vi "select energy.vi"(8 "Error In":errorcluster, 9 "List ROI in":dbl[][](array[numeric]), 10 "List Peak":string[][](table)=[["0", "0.738169", "8216.078017"], ["1", "1.925791", "11797.605609"], ["2", "2.296686", "59445.586632"], ["3", "2.951953", "7958.809520"], ["4", "3.301930", "5536.954047"], ["5", "3.693063", "592063.911968"], ["6", "4.012579", "88599.650063"], ["7", "5.456304", "6013.116723"], ["8", "5.905392", "7038.874622"], ["9", "6.404196", "22471.618393"], ["10", "7.049745", "8038.961303"], ["11", "7.336853", "5649.863203"], ["12", "7.978842", "3458.992769"], ["13", "8.617482", "7301.160509"], ["14", "9.554502", "1097.160220"], ["15", "10.523191", "20487.327187"], ["16", "11.054270", "2935.510385"], ["17", "11.234771", "2776.270069"], ["18", "12.573155", "28067.247871"], ["19", "13.048495", "7100.524309"], ["20", "13.060056", "7093.993228"], ["21", "13.100857", "7126.608473"], ["22", "13.283153", "7227.068614"], ["23", "14.060270", "10970.472713"], ["24", "14.659482", "8813.189447"], ["25", "15.701110", "4886.263831"], ["26", "16.589220", "151655.425908"], ["27", "17.295466", "73726.613413"], ["28", "18.547307", "16625.597400"], ["29", "19.386897", "11325.808412"], ["30", "23.791659", "1504.095156"], ["31", "24.239552", "1887.308691"], ["32", "24.942128", "13678.898904"]], 11 "Spectrum":cluster{"Channels":dbl[], "Intensity":dbl[]}[](graph)) -> (0 "Error Out":errorcluster, 1 "List ROI out":dbl[][](array[numeric]), 2 "Peak Position":cluster{"Array":dbl[], "Array":dbl[]}, 3 "Elements":string[][](table))   [LabVIEW 2023]
uses:
  <vilib>/Utility/miscctls.llb/LVRowAndColumnTypeDef.ctl
  06da3617-9ec4-42f1-9290-0e5eb46bbf30.vi
  84818e8e-7348-432d-a6d3-ef5b80d9228f.vi
  8a708491-6dff-4872-9c8c-723543562d7f.vi
  <vilib>/Utility/Data Type/Get Array Information.vi
  <vilib>/Utility/Data Type/Get Type Information.vi
  queue/Front Panel Message Queue.lvlib
panel:
  in  "list peak vs energy":bool
  out "reference list peak":refnum<vi>
  in  "Add":bool
  in  "ordinate":u16(ring) items=["Linear", "Logarithmic"]
  in  "doubt":bool
  in  "reset":bool
  out "List In":cluster{"Channels":dbl[], "Intensity":dbl[]}
  out "Data In":cluster{"Channels":dbl[], "Intensity":dbl[]}
  out "Element Position Peaks":dbl[][](array[numeric])
  out "Best Match":string[][](table)
  in  "exit":bool
  # "?"
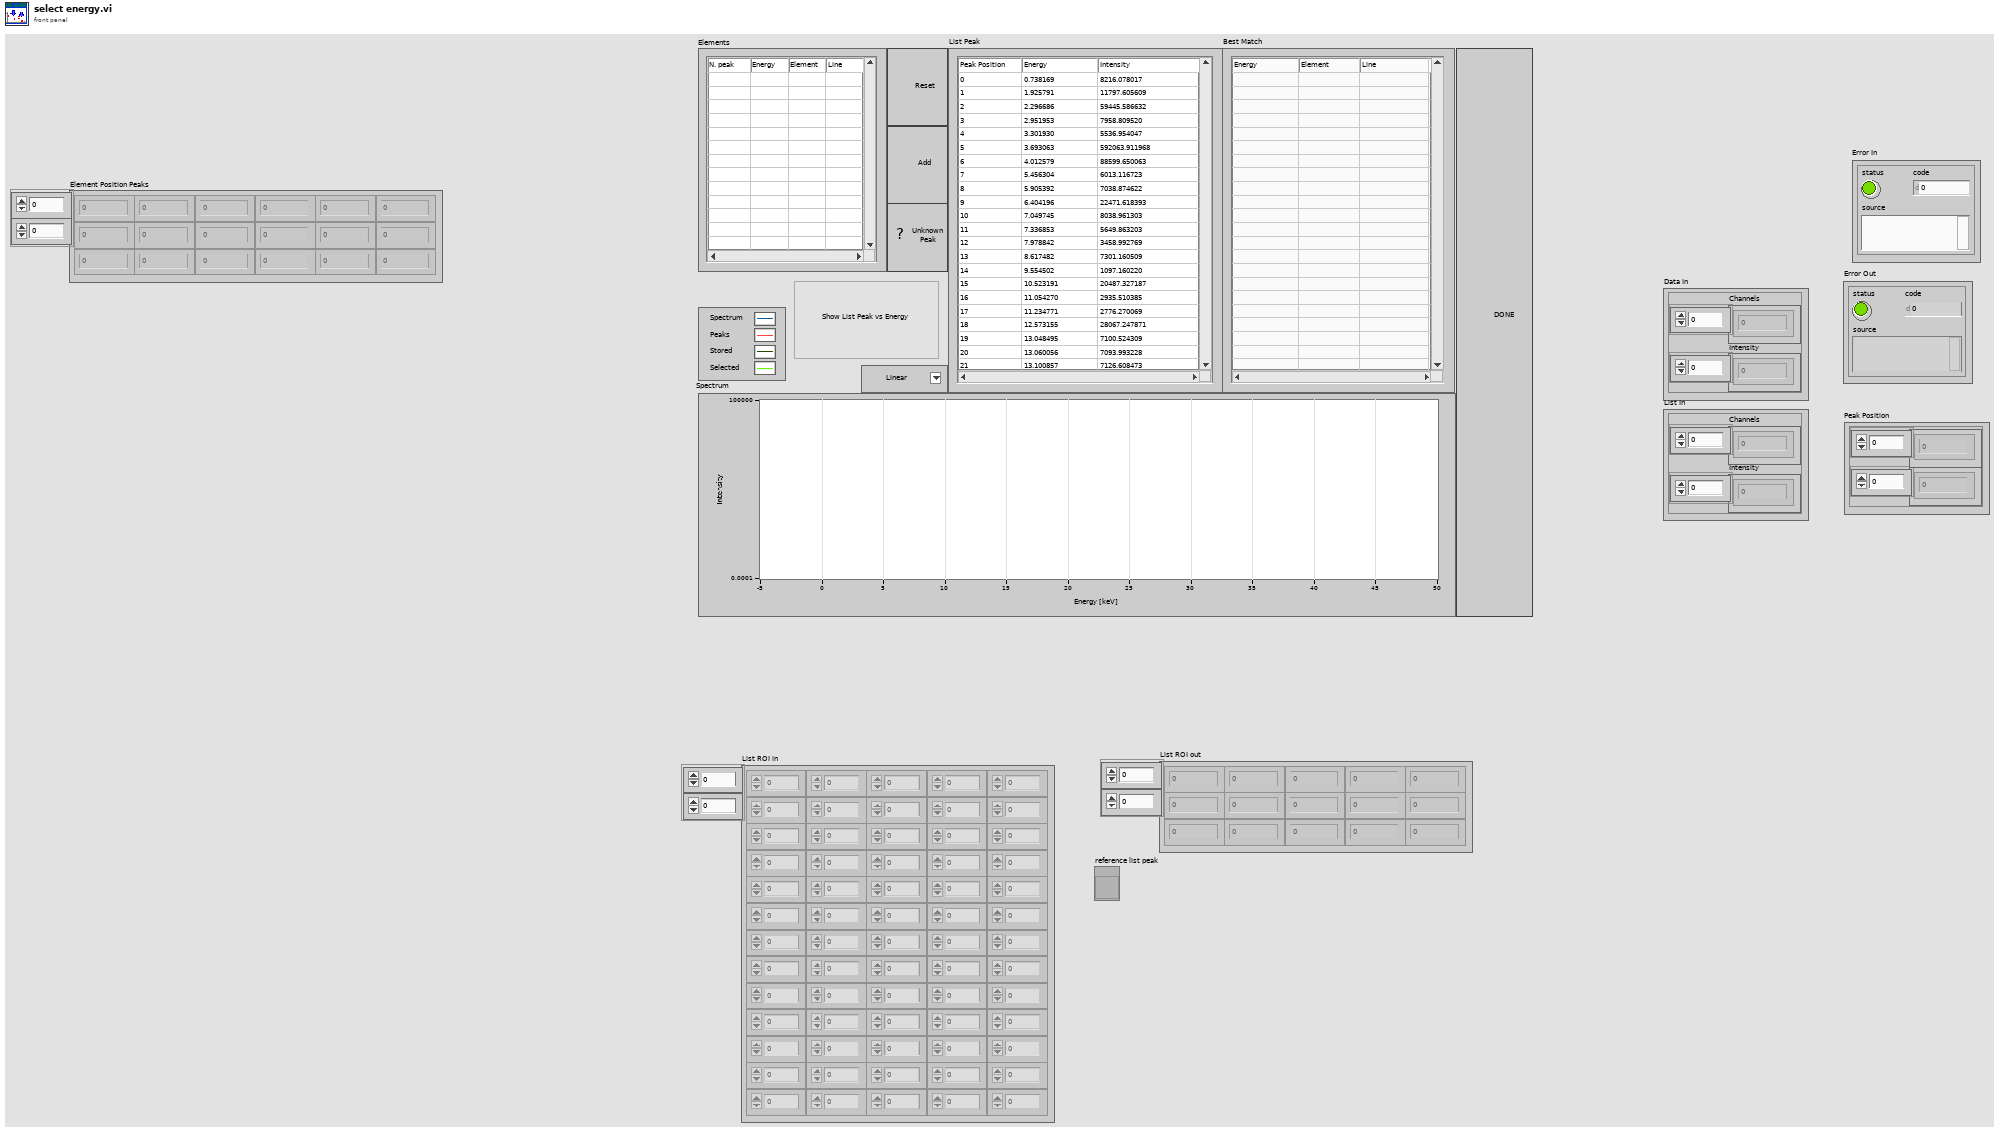
[diagram p1: front panel]
types:
  T1 = typedef "Front Panel Message Queue.lvlib/load Message Queues.ctl" = cluster{"Main":refnum<queue>}
  T2 = enum32{"Invalid", "Standard", "Closed", "Hidden", "Minimized", "Maximized"}
  T3 = typedef "LVRowAndColumnTypeDef.ctl" = cluster{"Row":i32, "Column":i32}
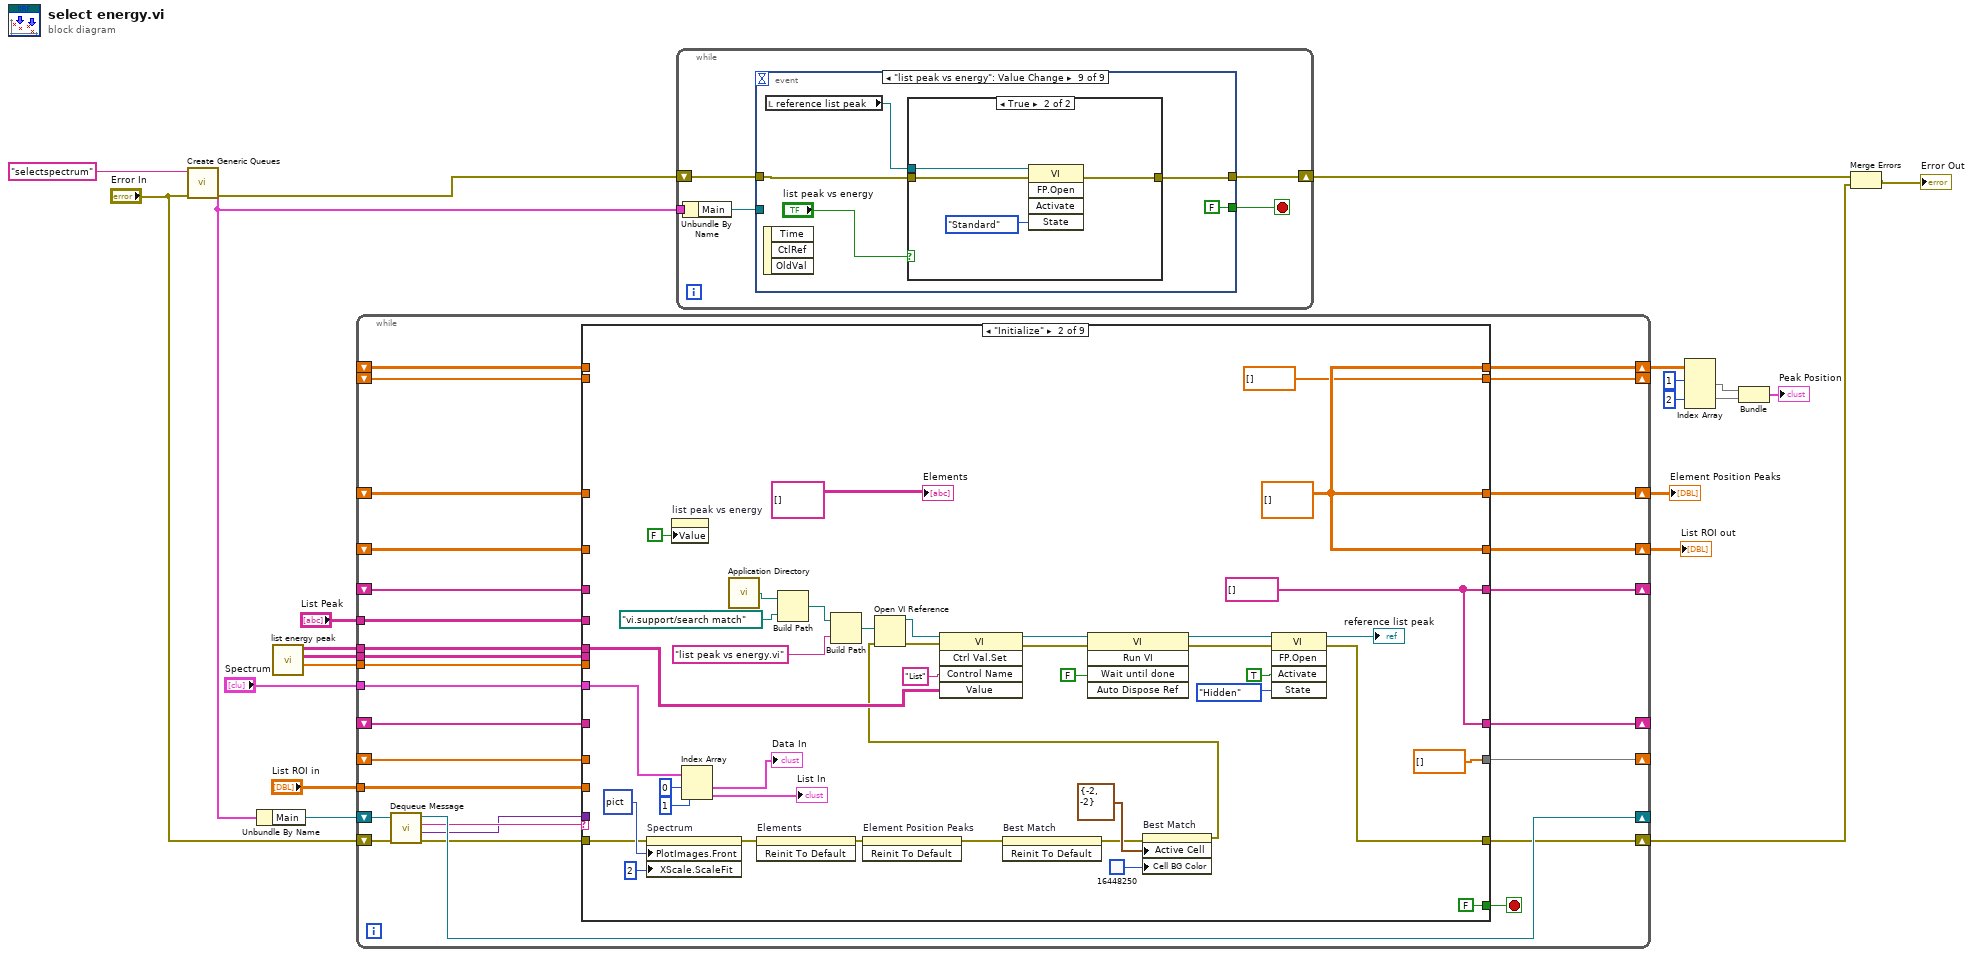
[diagram p0: block diagram]
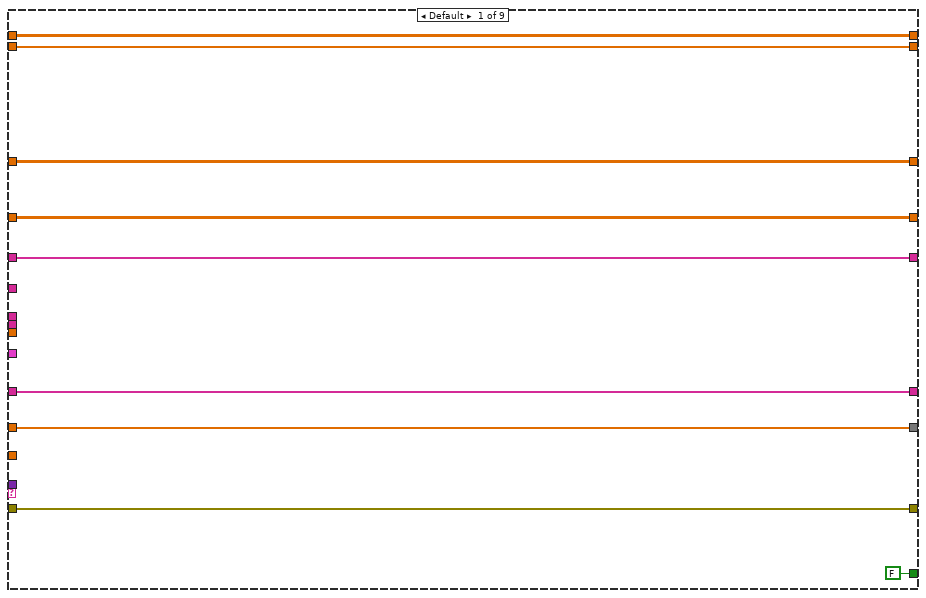
[diagram p2: hidden frame]
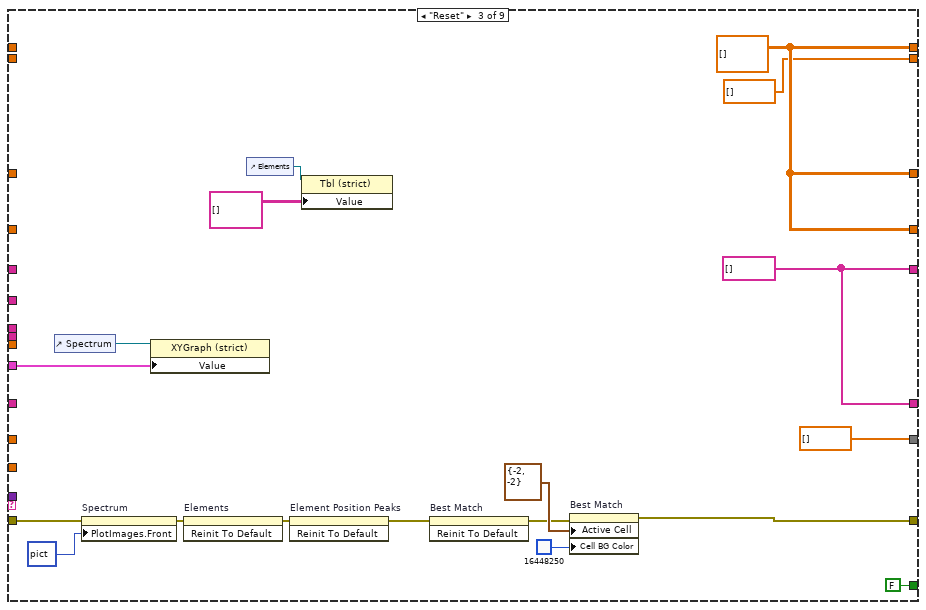
[diagram p3: hidden frame]
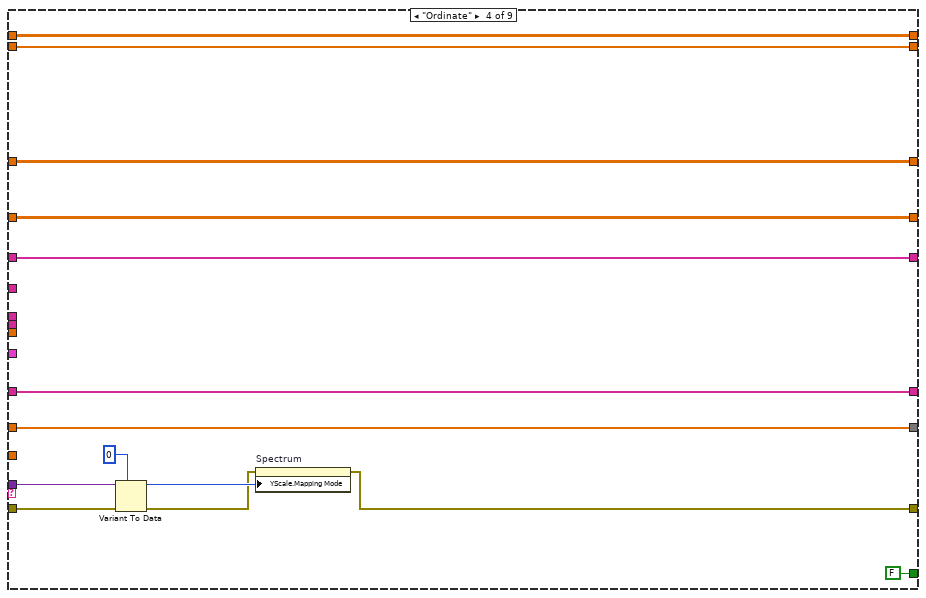
[diagram p4: hidden frame]
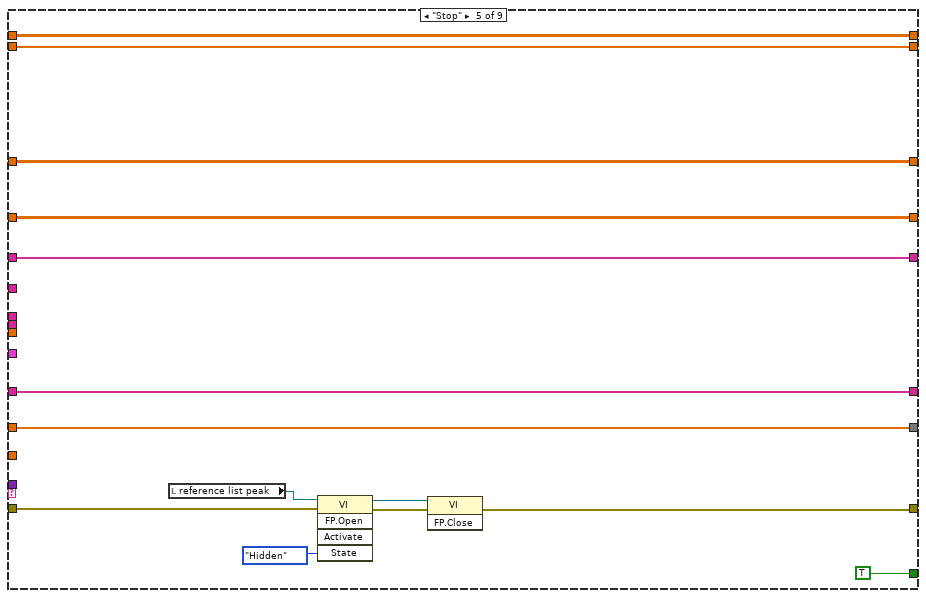
[diagram p5: hidden frame]
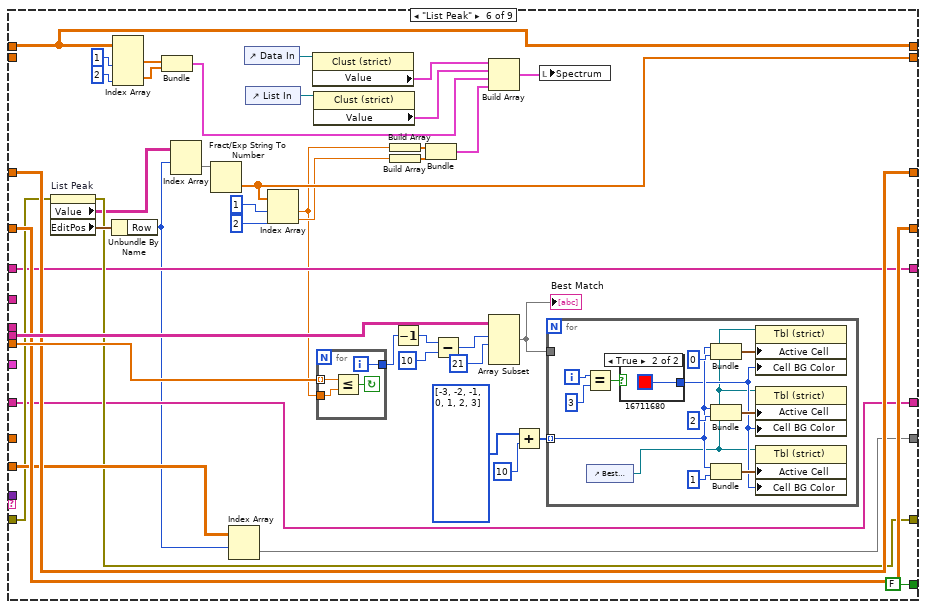
[diagram p6: hidden frame]
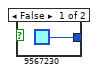
[diagram p7: hidden frame]
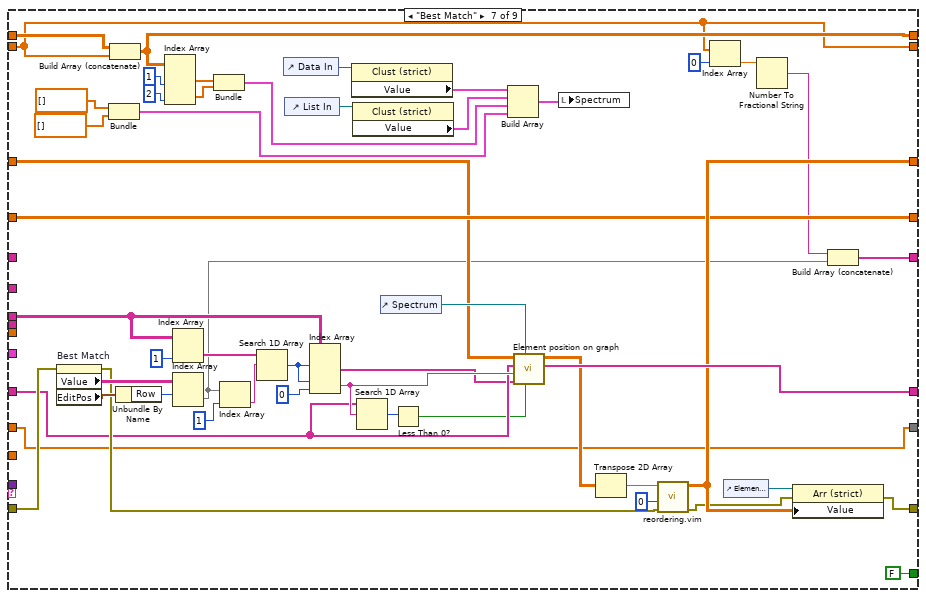
[diagram p8: hidden frame]
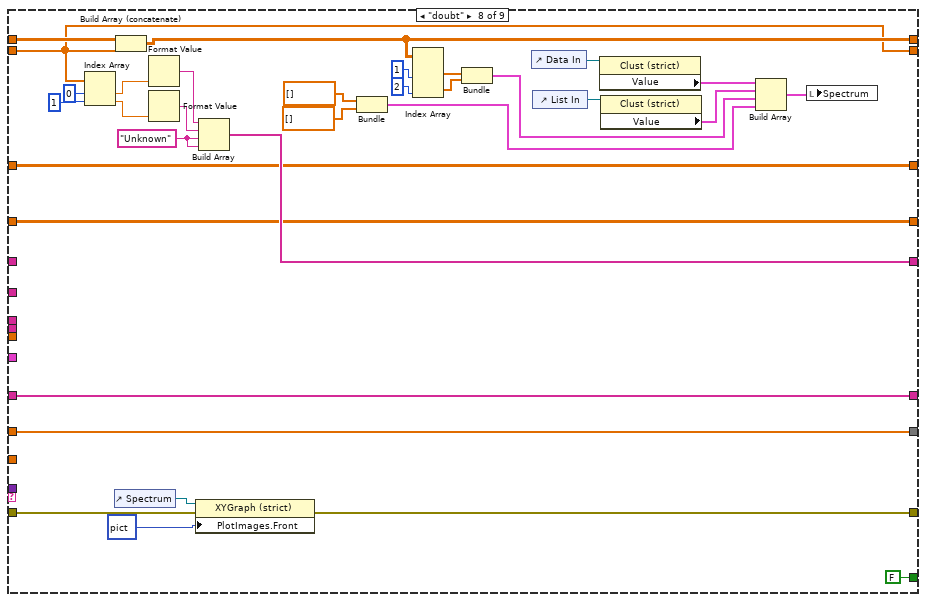
[diagram p9: hidden frame]
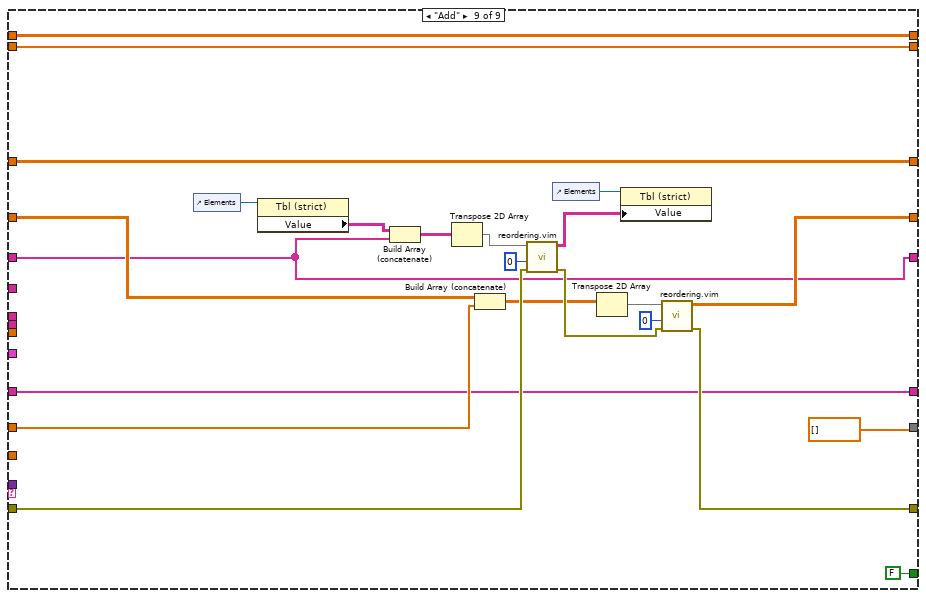
[diagram p10: hidden frame]
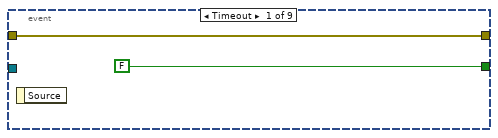
[diagram p11: hidden frame]
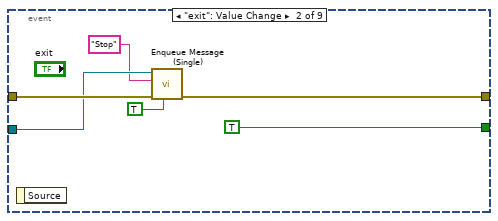
[diagram p12: hidden frame]
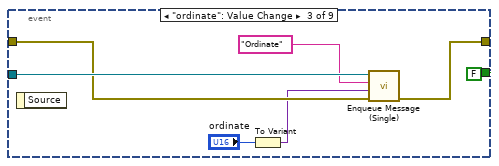
[diagram p13: hidden frame]
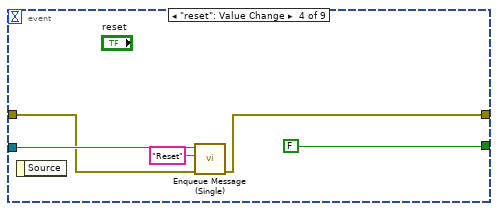
[diagram p14: hidden frame]
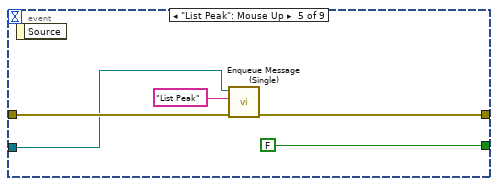
[diagram p15: hidden frame]
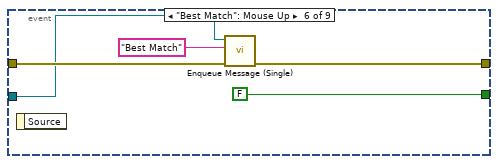
[diagram p16: hidden frame]
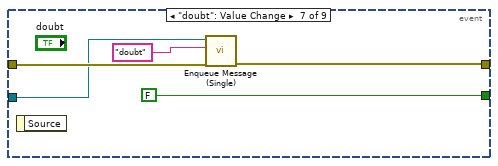
[diagram p17: hidden frame]
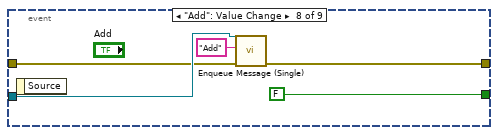
[diagram p18: hidden frame]
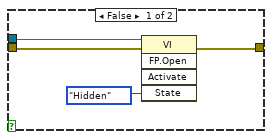
[diagram p19: hidden frame]
diagram:
  n1 = call "Create Generic Queues.vi"("error in (no error)"="Error In", "name"="selectspectrum") -> ("error out"=w21:errorcluster, "Message Queues"=w14:T1)  [unwired: 8 in]
  n2 = Unbundle By Name(w14) -> ("Main"=w19:refnum<queue>)
  n3 = call "list energy peak.vi"() -> ("Energies Ordered"=w15:dbl[], "List Ordered"=w16:string[][], "List"=w17:string[][])  [unwired: 6 in, 3 out]
  n4 = while {
    shift-right: [w45] -> w2
    shift-left: "Error In" -> [w50]
    shift-right: [w48] -> _
    shift-left: w19 -> [w49]
    tunnel: "Spectrum" -> [w47]
    tunnel: w17 -> [w23]
    tunnel: w16 -> [w25]
    tunnel: w15 -> [w26]
    shift-right: [w41] -> _
    shift-left: _ -> [w40]
    shift-right: [w39] -> w10
    shift-left: _ -> [w38]
    shift-right: [w37] -> w11
    shift-left: _ -> [w32]
    shift-right: [w36] -> w5
    shift-left: _ -> [w33]
    shift-right: [w35] -> _
    shift-left: _ -> [w34]
    shift-right: [w31] -> _
    shift-left: _ -> [w28]
    shift-right: [w30] -> _
    shift-left: _ -> [w29]
    tunnel: "List Peak" -> [w27]
    tunnel: "List ROI in" -> [w24]
    stop <- w43 stop-if-true
    n5 = call "Dequeue Message.vi"("error in (no error)"=w50, "Message Queue"=w49) -> ("error out"=w46:errorcluster, "Message Data"=w42:variant, "Message"=w44:string, "dup Message Queue"=w48:refnum<queue>)  [unwired: 5 in, 1 out]
    n6 = case shown="\"Initialize\"" w44 {
      tunnel: w46 -> [w58 w92 w110 w130 w136 w158 w240 w279 w305]
      tunnel: w47 -> [_ w89 w106 _ _ _ _ _ _]
      tunnel: [w58 w69 w109 w127 w132 w159 w219 w277 w301] -> w45
      tunnel: [FALSE FALSE FALSE FALSE TRUE FALSE FALSE FALSE FALSE] -> w43
      tunnel: w42 -> [_ _ _ w125 _ _ _ _ _]
      tunnel: [w57 dbl[] [] dbl[] [] w124 w144 w152 w228 w260 w292] -> w41
      tunnel: w40 -> [w57 _ _ w124 w144 _ w228 w260 w292]
      tunnel: [w53 w85 w105 w123 w143 w177 w253 w261 w291] -> w39
      tunnel: w38 -> [w53 _ _ w123 w143 w177 w256 w289 w291]
      tunnel: [w54 w85 w105 w122 w142 w166 w221 w273 w293] -> w37
      tunnel: [w55 w85 w105 w121 w141 w167 w216 w274 w298] -> w36
      tunnel: [w56 dbl[] [] dbl[] [] w120 w140 w164 w217 w276 dbl[] []] -> w35
      tunnel: w34 -> [w56 _ _ w120 w140 _ w217 w276 w299]
      tunnel: w33 -> [w55 _ _ w121 w141 w167 w216 w274 w297]
      tunnel: w32 -> [w54 _ _ w122 w142 w166 w215 w273 w293]
      tunnel: [w52 w83 w101 w119 w139 w157 w229 w281 w294] -> w31
      tunnel: [w51 w83 w101 w118 w138 w156 w227 w275 w295] -> w30
      tunnel: w29 -> [w51 _ _ w118 w138 w156 w213 w275 w295]
      tunnel: w28 -> [w52 _ _ w119 w139 w157 _ _ w294]
      tunnel: w27 -> [_ _ _ _ _ _ _ _ _]
      tunnel: w26 -> [_ _ _ _ _ w174 _ _ _]
      tunnel: w25 -> [_ _ _ _ _ w168 _ _ _]
      tunnel: w24 -> [_ _ _ _ _ w165 _ _ _]
      tunnel: w23 -> [_ w72 _ _ _ _ w235 _ _]
      frame Default {
      }
      frame "Initialize" {
        w83 = string[] [] ("Value")
        w85 = dbl[][] []
        n7 = property on="Spectrum" class="XYGraph (strict)"(error in=w92, "PlotImages.Front"=picture data[5B] ("line to place"), "XScale.ScaleFit"=u8 2 ("X Scale.Scale Fit")) -> (error out=w99:errorcluster)  [unwired: 1 in, 1 out]
        n8 = property on="list peak vs energy" class="Bool (strict)"("Value"=FALSE ("list peak")) -> ()  [unwired: 2 in, 2 out]
        n9 = Index Array(array=w89, index #1=0 ("index"), index #2=1 ("index")) -> (element #1=→"Data In":cluster{"Channels":dbl[], "Intensity":dbl[]}, element #2=→"List In":cluster{"Channels":dbl[], "Intensity":dbl[]})
        n10 = call <vilib>:"Application Directory.vi"() -> ("Application Directory"=w79:path)
        n11 = invoke on="Elements" class="Tbl (strict)" method="Reinit To Default"(error in=w99) -> (error out=w93:errorcluster)  [unwired: 2 in, 2 out]
        n12 = Build Path(base path=w79, name or relative path=path "vi.support/search match") -> (appended path=w74:path)
        n13 = Build Path(base path=w74, name or relative path="list peak vs energy.vi") -> (appended path=w76:path)
        n14 = invoke on="Element Position Peaks" class="Arr (strict)" method="Reinit To Default"(error in=w93) -> (error out=w97:errorcluster)  [unwired: 2 in, 2 out]
        n15 = invoke on="Best Match" class="Tbl (strict)" method="Reinit To Default"(error in=w97) -> (error out=w94:errorcluster)  [unwired: 2 in, 2 out]
        n16 = property on="Best Match" class="Tbl (strict)"(error in=w94, "Active Cell"=T3 {"Row"=-2, "Column"=-2} ("Active Cell:Active Cell"), "Cell BG Color"=u32 16448250) -> (error out=w71:errorcluster)  [unwired: 1 in, 1 out]
        n17 = Open VI Reference(vi path=w76, error in (no error)=w71) -> (vi reference=w66:refnum<vi>, error out=w65:errorcluster)  [unwired: 4 in]
        n18 = invoke class="VI" method="Ctrl Val.Set"(reference=w66, error in=w65, "Control Name"="List", "Value"=w72) -> (reference out=w64:refnum<vi>, error out=w63:errorcluster)  [unwired: 1 in, 3 out]
        n19 = invoke class="VI" method="Run VI"(reference=w64, error in=w63, "Wait until done"=FALSE ("Wait Until Done")) -> (reference out=w61:refnum<vi>, error out=w62:errorcluster)  [unwired: 2 in, 3 out]
        n20 = invoke class="VI" method="FP.Open"(reference=w61, error in=w62, "Activate"=TRUE ("Activate?"), "State"=T2."Hidden") -> (reference out=→"reference list peak":refnum<vi>, error out=w69:errorcluster)  [unwired: 1 in, 3 out]
        "Elements" <- string[][] [] ("Data Out")
      }
      frame "Reset" {
        w101 = string[] [] ("Value")
        w105 = dbl[][] []
        n21 = control-ref of="Spectrum"() -> (w107:refnum<vi>)
        n22 = property on="Spectrum" class="XYGraph (strict)"(error in=w110, "PlotImages.Front"=picture data[5B] ("line to place")) -> (error out=w117:errorcluster)  [unwired: 1 in, 1 out]
        n23 = property class="XYGraph (strict)"(reference=w107, "Value"=w106) -> ()  [unwired: 1 in, 2 out]
        n24 = invoke on="Elements" class="Tbl (strict)" method="Reinit To Default"(error in=w117) -> (error out=w111:errorcluster)  [unwired: 2 in, 2 out]
        n25 = control-ref of="Elements"() -> (w103:refnum<vi>)
        n26 = invoke on="Element Position Peaks" class="Arr (strict)" method="Reinit To Default"(error in=w111) -> (error out=w115:errorcluster)  [unwired: 2 in, 2 out]
        n27 = property class="Tbl (strict)"(reference=w103, "Value"=string[][] [] ("Data Out")) -> ()  [unwired: 1 in, 2 out]
        n28 = invoke on="Best Match" class="Tbl (strict)" method="Reinit To Default"(error in=w115) -> (error out=w112:errorcluster)  [unwired: 2 in, 2 out]
        n29 = property on="Best Match" class="Tbl (strict)"(error in=w112, "Active Cell"=T3 {"Row"=-2, "Column"=-2} ("Active Cell:Active Cell"), "Cell BG Color"=u32 16448250) -> (error out=w109:errorcluster)  [unwired: 1 in, 1 out]
      }
      frame "Ordinate" {
        n30 = Variant To Data(error in=w130, type=u16 0, Variant=w125) -> (data=w128:u16, error out=w126:errorcluster)
        n31 = property on="Spectrum" class="XYGraph (strict)"(error in=w126, "YScale.Mapping Mode"=w128) -> (error out=w127:errorcluster)  [unwired: 1 in, 1 out]
      }
      frame "Stop" {
        n32 = local read "reference list peak"() -> (w135:refnum<vi>)
        n33 = invoke class="VI" method="FP.Open"(reference=w135, error in=w136, "State"=T2."Hidden") -> (reference out=w134:refnum<vi>, error out=w133:errorcluster)  [unwired: 2 in, 3 out]
        n34 = invoke class="VI" method="FP.Close"(reference=w134, error in=w133) -> (error out=w132:errorcluster)  [unwired: 1 in, 2 out]
      }
      frame "List Peak" {
        n35 = property on="List Peak" class="Tbl (strict)"(error in=w158) -> (error out=w159:errorcluster, "Value"=w155:string[][], "EditPos"=w176:T3)  [unwired: 1 in, 1 out]
        n36 = Unbundle By Name(w176) -> ("Row"=w154:i32)
        n37 = Index Array(array=w177, index (col) #1=1 ("index (row)"), index (col) #2=2 ("index (row)")) -> (element #1=w187:dbl[], element #2=w186:dbl[])  [unwired: 2 in]
        n38 = Bundle(w187, w186) -> (w178:cluster{dbl[], dbl[]})  [unwired: 1 in]
        n39 = Index Array(array=w155, index (row)=w154) -> (element=w153:string[])  [unwired: 1 in]
        n40 = Fract/Exp String To Number(string=w153) -> (number=w152:dbl[])  [unwired: 3 in, 1 out]
        n41 = Index Array(array=w165, index (row)=w154) -> (element=w164:dbl[])  [unwired: 1 in]
        n42 = control-ref of="Data In"() -> (w182:refnum<vi>)
        n43 = control-ref of="List In"() -> (w181:refnum<vi>)
        n44 = Index Array(array=w152, index #1=1 ("index"), index #2=2 ("index")) -> (element #1=w148:dbl, element #2=w149:dbl)
        n45 = property class="Clust (strict)"(reference=w182) -> ("Value"=w180:cluster{"Channels":dbl[], "Intensity":dbl[]})  [unwired: 1 in, 2 out]
        n46 = property class="Clust (strict)"(reference=w181) -> ("Value"=w179:cluster{"Channels":dbl[], "Intensity":dbl[]})  [unwired: 1 in, 2 out]
        n47 = for {
          tunnel: w174 -> [w206] mode=indexing
          tunnel: w148 -> [w205]
          tunnel: [w203] -> w173
          i -> [w203]
          stop <- w204 continue-if-true
          n48 = Less Or Equal?(x=w206, y=w205) -> (x <= y?=w204:bool)
        }
        n49 = Build Array(w148) -> (w185:dbl[])
        n50 = Build Array(w149) -> (w184:dbl[])
        n51 = Decrement(x=w173) -> (x-1=w171:i32)
        n52 = Bundle(w185, w184) -> (w175:cluster{dbl[], dbl[]})  [unwired: 1 in]
        n53 = Subtract(x=w171, y=10) -> (x-y=w169:i32)
        n54 = Build Array(w180, w179, w178, w175) -> (w183:cluster{"Channels":dbl[], "Intensity":dbl[]}[])
        n55 = Array Subset(array=w168, index (row)=w169, length (row)=21 ("length")) -> (w160:string[][])  [unwired: 2 in]
        "Best Match" <- w160
        n56 = Add(x=i32[] [-3, -2, -1, 0, 1, 2, 3], y=10) -> (x+y=w163:i32[])
        n57 = local write "Spectrum"(w183) -> ()
        n58 = for {
          tunnel: w163 -> [w192] mode=indexing
          tunnel: w160 -> [_]
          i -> [w200]
          n59 = Equal?(x=w200, y=3) -> (x = y?=w198:bool)
          n60 = control-ref of="Best Match"() -> (w189:refnum<vi>)
          n61 = case shown="True" w198 {
            tunnel: [u32 9567230 u32 16711680] -> w190
            frame False {
            }
            frame True {
            }
          }
          n62 = Bundle(w192, 0) -> (w191:cluster{i32, i32})  [unwired: 1 in]
          n63 = Bundle(w192, 2) -> (w194:cluster{i32, i32})  [unwired: 1 in]
          n64 = Bundle(w192, 1) -> (w195:cluster{i32, i32})  [unwired: 1 in]
          n65 = property on="Property Node" class="Tbl (strict)"(reference=w189, "Active Cell"=w191, "Cell BG Color"=w190) -> ()  [unwired: 1 in, 2 out]
          n66 = property on="Property Node" class="Tbl (strict)"(reference=w189, "Active Cell"=w194, "Cell BG Color"=w190) -> ()  [unwired: 1 in, 2 out]
          n67 = property on="Property Node" class="Tbl (strict)"(reference=w189, "Active Cell"=w195, "Cell BG Color"=w190) -> ()  [unwired: 1 in, 2 out]
        }
      }
      frame "Best Match" {
        n68 = property on="Best Match" class="Tbl (strict)"(error in=w240) -> (error out=w224:errorcluster, "Value"=w242:string[][], "EditPos"=w241:T3)  [unwired: 1 in, 1 out]
        n69 = Bundle(dbl[] [], dbl[] []) -> (w244:cluster{dbl[], dbl[]})  [unwired: 1 in]
        n70 = Build Array (concatenate)(w256, w228) -> (w253:dbl[][])
        n71 = Unbundle By Name(w241) -> ("Row"=w243:i32)
        n72 = Index Array(array=w253, index (col) #1=1 ("index (row)"), index (col) #2=2 ("index (row)")) -> (element #1=w255:dbl[], element #2=w254:dbl[])  [unwired: 2 in]
        n73 = Index Array(array=w235, index (col)=1 ("disabled index (col)")) -> (element=w238:string[])  [unwired: 1 in]
        n74 = Index Array(array=w242, index (row)=w243) -> (element=w210:string[])  [unwired: 1 in]
        n75 = Bundle(w255, w254) -> (w247:cluster{dbl[], dbl[]})  [unwired: 1 in]
        n76 = Index Array(array=w210, index=1) -> (element=w232:string)
        n77 = Search 1D Array(1D array=w238, element=w232) -> (index of element=w236:i32)  [unwired: 1 in]
        n78 = control-ref of="Data In"() -> (w250:refnum<vi>)
        n79 = control-ref of="List In"() -> (w249:refnum<vi>)
        n80 = Index Array(array=w235, index (row) #1=w236, index (row) #2=w236, index (col) #2=0 ("disabled index (col)")) -> (element #1=w212:string[], element #2=w214:string)  [unwired: 1 in]
        n81 = property class="Clust (strict)"(reference=w250) -> ("Value"=w248:cluster{"Channels":dbl[], "Intensity":dbl[]})  [unwired: 1 in, 2 out]
        n82 = property class="Clust (strict)"(reference=w249) -> ("Value"=w252:cluster{"Channels":dbl[], "Intensity":dbl[]})  [unwired: 1 in, 2 out]
        n83 = Search 1D Array(1D array=w213, element=w214) -> (index of element=w234:i32)  [unwired: 1 in]
        n84 = control-ref of="Spectrum"() -> (w218:refnum<vi>)
        n85 = Less Than 0?(x=w234) -> (x < 0?=w211:bool)
        n86 = Build Array(w248, w252, w247, w244) -> (w251:cluster{"Channels":dbl[], "Intensity":dbl[]}[])
        n87 = call "Element position on graph.vi"("Check Element"=w211, "Spectrum"=w218, "List"=w212, "String"=w214, "List Elements in"=w213, "Elements Position Peaks in"=w215) -> ("List Elements out"=w227:string[], "Element Position Peaks out"=w223:dbl[][])  [unwired: 4 in]
        n88 = local write "Spectrum"(w251) -> ()
        n89 = Transpose 2D Array(2D array=w223) -> (transposed array=w225:dbl[][])
        n90 = call "reordering.vim"("error in (no error)"=w224, "Row to Reorder"=0, "Data In"=w225) -> ("Error Out"=w220:errorcluster, "Data Out"=w221:dbl[][])  [unwired: 7 in]
        n91 = Index Array(array=w228, index=0) -> (element=w231:dbl)
        n92 = control-ref of="Element Position Peaks"() -> (w222:refnum<vi>)
        n93 = Number To Fractional String(number=w231) -> (F-format string=w209:string)  [unwired: 3 in]
        n94 = property class="Arr (strict)"(reference=w222, error in=w220, "Value"=w221) -> (error out=w219:errorcluster)  [unwired: 1 out]
        n95 = Build Array (concatenate)(w209, w210) -> (w229:string[])
      }
      frame "doubt" {
        w282 = "Unknown"
        n96 = Index Array(array=w260, index #1=0 ("index"), index #2=1 ("index")) -> (element #1=w286:dbl, element #2=w285:dbl)
        n97 = control-ref of="Spectrum"() -> (w280:refnum<vi>)
        n98 = Build Array (concatenate)(w289, w260) -> (w261:dbl[][])
        n99 = Format Value(value (0)=w286) -> (output string=w284:string)  [unwired: 2 in]
        n100 = Format Value(value (0)=w285) -> (output string=w283:string)  [unwired: 2 in]
        n101 = property class="XYGraph (strict)"(reference=w280, error in=w279, "PlotImages.Front"=picture data[5B] ("line to place")) -> (error out=w277:errorcluster)  [unwired: 1 out]
        n102 = Build Array(w284, w283, w282, w282) -> (w281:string[])
        n103 = Bundle(dbl[] [], dbl[] []) -> (w272:cluster{dbl[], dbl[]})  [unwired: 1 in]
        n104 = Index Array(array=w261, index (col) #1=1 ("index (row)"), index (col) #2=2 ("index (row)")) -> (element #1=w271:dbl[], element #2=w270:dbl[])  [unwired: 2 in]
        n105 = Bundle(w271, w270) -> (w264:cluster{dbl[], dbl[]})  [unwired: 1 in]
        n106 = control-ref of="Data In"() -> (w267:refnum<vi>)
        n107 = control-ref of="List In"() -> (w266:refnum<vi>)
        n108 = property class="Clust (strict)"(reference=w267) -> ("Value"=w265:cluster{"Channels":dbl[], "Intensity":dbl[]})  [unwired: 1 in, 2 out]
        n109 = property class="Clust (strict)"(reference=w266) -> ("Value"=w269:cluster{"Channels":dbl[], "Intensity":dbl[]})  [unwired: 1 in, 2 out]
        n110 = Build Array(w265, w269, w264, w272) -> (w268:cluster{"Channels":dbl[], "Intensity":dbl[]}[])
        n111 = local write "Spectrum"(w268) -> ()
      }
      frame "Add" {
        n112 = control-ref of="Elements"() -> (w309:refnum<vi>)
        n113 = property class="Tbl (strict)"(reference=w309) -> ("Value"=w306:string[][])  [unwired: 1 in, 2 out]
        n114 = Build Array (concatenate)(w306, w294) -> (w310:string[][])
        n115 = Transpose 2D Array(2D array=w310) -> (transposed array=w311:string[][])
        n116 = Build Array (concatenate)(w297, w299) -> (w300:dbl[][])
        n117 = call "reordering.vim"("error in (no error)"=w305, "Row to Reorder"=0, "Data In"=w311) -> ("Error Out"=w302:errorcluster, "Data Out"=w307:string[][])  [unwired: 7 in]
        n118 = control-ref of="Elements"() -> (w308:refnum<vi>)
        n119 = Transpose 2D Array(2D array=w300) -> (transposed array=w303:dbl[][])
        n120 = property class="Tbl (strict)"(reference=w308, "Value"=w307) -> ()  [unwired: 1 in, 2 out]
        n121 = call "reordering.vim"("error in (no error)"=w302, "Row to Reorder"=0, "Data In"=w303) -> ("Error Out"=w301:errorcluster, "Data Out"=w298:dbl[][])  [unwired: 7 in]
      }
    }
  }
  "Element Position Peaks" <- w11
  "List ROI out" <- w5
  n122 = while {
    shift-right: [w317] -> w4
    shift-left: w21 -> [w316]
    tunnel: w14 -> [w315]
    stop <- w318 stop-if-true
    n123 = Unbundle By Name(w315) -> ("Main"=w314:refnum<queue>)
    n124 = event shown="[8] \"list peak vs energy\": Value Change" {
      selector: _ -> [_ _ _ _ _ _ _ _ _]
      dyn-events: _ -> [_ _ _ _ _ _ _ _ _]
      timeout: _ -> [_ _ _ _ _ _ _ _ _]
      tunnel: [FALSE ("Stop Button") TRUE ("Stop Button") FALSE ("Stop Button") FALSE ("Stop Button") FALSE ("Stop Button") FALSE ("Stop Button") FALSE ("Stop Button") FALSE ("Stop Button") FALSE ("Stop Button")] -> w318
      tunnel: [w319 w322 w330 w336 w341 w345 w350 w354 w359] -> w317
      tunnel: w316 -> [w319 w325 w331 w335 w340 w346 w351 w355 w360]
      tunnel: w314 -> [_ w324 w332 w337 w339 w344 w349 w356 _]
      event Timeout {
        n125 = event-data() -> ()  [unwired: 1 in, 1 out]
      }
      event "exit": Value Change {
        n126 = event-data() -> ()  [unwired: 1 in, 1 out]
        n127 = call "Enqueue Message (Single).vi"("Priority Message? (F)"=TRUE, "error in (no error)"=w325, "Message"="Stop", "Message Queue"=w324) -> ("error out"=w322:errorcluster)  [unwired: 6 in, 1 out]
      }
      event "ordinate": Value Change {
        n128 = event-data() -> ()  [unwired: 1 in, 1 out]
        n129 = To Variant(anything="ordinate") -> (Variant=w327:variant)
        n130 = call "Enqueue Message (Single).vi"("error in (no error)"=w331, "Message Data"=w327, "Message"="Ordinate", "Message Queue"=w332) -> ("error out"=w330:errorcluster)  [unwired: 6 in, 1 out]
      }
      event "reset": Value Change {
        n131 = event-data() -> ()  [unwired: 1 in, 1 out]
        n132 = call "Enqueue Message (Single).vi"("error in (no error)"=w335, "Message"="Reset", "Message Queue"=w337) -> ("error out"=w336:errorcluster)  [unwired: 7 in, 1 out]
      }
      event "List Peak": Mouse Up {
        n133 = event-data() -> ()  [unwired: 1 in, 1 out]
        n134 = call "Enqueue Message (Single).vi"("error in (no error)"=w340, "Message"="List Peak", "Message Queue"=w339) -> ("error out"=w341:errorcluster)  [unwired: 7 in, 1 out]
      }
      event "Best Match": Mouse Up {
        n135 = event-data() -> ()  [unwired: 1 in, 1 out]
        n136 = call "Enqueue Message (Single).vi"("error in (no error)"=w346, "Message"="Best Match", "Message Queue"=w344) -> ("error out"=w345:errorcluster)  [unwired: 7 in, 1 out]
      }
      event "doubt": Value Change {
        n137 = event-data() -> ()  [unwired: 1 in, 1 out]
        n138 = call "Enqueue Message (Single).vi"("error in (no error)"=w351, "Message"="doubt", "Message Queue"=w349) -> ("error out"=w350:errorcluster)  [unwired: 7 in, 1 out]
      }
      event "Add": Value Change {
        n139 = event-data() -> ()  [unwired: 1 in, 1 out]
        n140 = call "Enqueue Message (Single).vi"("error in (no error)"=w355, "Message"="Add", "Message Queue"=w356) -> ("error out"=w354:errorcluster)  [unwired: 7 in, 1 out]
      }
      event "list peak vs energy": Value Change {
        n141 = event-data() -> ()  [unwired: 1 in, 3 out]
        n142 = local read "reference list peak"() -> (w361:refnum<vi>)
        n143 = case shown="True" "list peak vs energy" {
          tunnel: w361 -> [w365 w371]
          tunnel: w360 -> [w366 w370]
          tunnel: [w364 w369] -> w359
          frame False {
            n144 = invoke class="VI" method="FP.Open"(reference=w365, error in=w366, "State"=T2."Hidden") -> (error out=w364:errorcluster)  [unwired: 2 in, 4 out]
          }
          frame True {
            n145 = invoke class="VI" method="FP.Open"(reference=w371, error in=w370, "State"=T2."Standard") -> (error out=w369:errorcluster)  [unwired: 2 in, 4 out]
          }
        }
      }
    }
  }
  n146 = Index Array(array=w10, index (row) #1=1 ("index (row)"), index (row) #2=2 ("index (row)")) -> (element #1=w7:dbl[], element #2=w6:dbl[])  [unwired: 2 in]
  n147 = Bundle(w7, w6) -> (→"Peak Position":cluster{dbl[], dbl[]})  [unwired: 1 in]
  n148 = Merge Errors(w4, w2) -> (→"Error Out":errorcluster)
